vi "Weigth-Voltage.vi"() -> ()   [LabVIEW 2015]
uses:
  <vilib>/Utility/error.llb/DialogType.ctl
  <vilib>/DAQmx/read.llb/DAQmx Read (Analog DBL 1Chan 1Samp).vi
  <vilib>/DAQmx/create/channels.llb/DAQmx Create Channel (AI-Voltage-Basic).vi
  <vilib>/DAQmx/miscellaneous.llb/DAQmx Fill In Error Info.vi
panel:
  out "Peso[g]":dbl
  out "Waveform Chart":dbl(graph)
  out "Vi":dbl=0.7398038924745398 format="%0.2f"
  in  "stop":bool
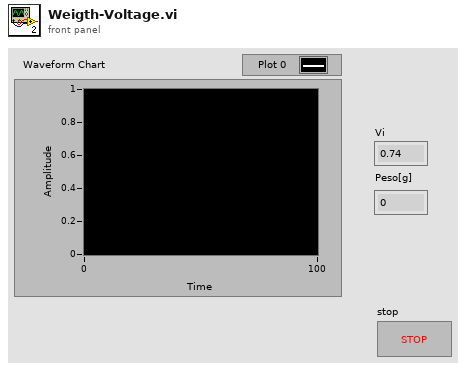
[diagram p1: front panel]
types:
  T1 = typedef "DialogType.ctl" = u16
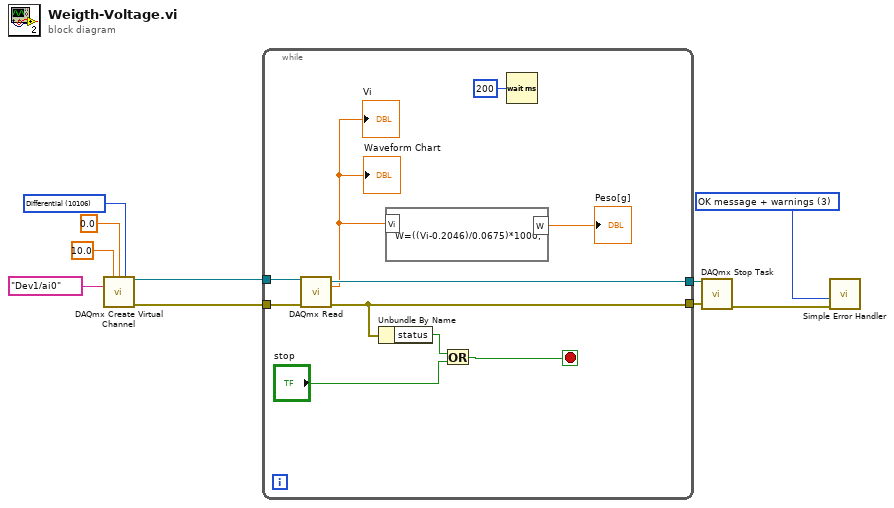
[diagram p0: block diagram]
diagram:
  w1 = 10106 items=["Default"=-1, "RSE"=10083, "NRSE"=10078, "Differential"=10106, "Pseudodifferential"=12529] ("input terminal configuration")
  w2 = T1 3 items=["no dialog", "OK message", "continue or stop message", "OK message + warnings", "continue/stop + warnings"] ("type of dialog (OK msg:1)")
  n1 = call-poly <vilib>:"DAQmx Create Virtual Channel.vi"("maximum value"=10.0, "minimum value"=0.0, "input terminal configuration"=w1, "physical channels"=tag "Dev1/ai0") -> ("task out"=w7:refnum<k21>, "error out"=w6:errorcluster)  [unwired: 10 in]
  n2 = while {
    tunnel: w7 -> [w20]
    tunnel: w6 -> [w19]
    tunnel: [w18] -> w5
    tunnel: [w14] -> w4
    stop <- w15 stop-if-true
    n3 = call-poly <vilib>:"DAQmx Read.vi"("task/channels in"=w20, "error in"=w19) -> ("task out"=w14:refnum<k21>, "data"=w12:dbl, "error out"=w18:errorcluster)  [unwired: 11 in]
    "Vi" <- w12
    "Waveform Chart" <- w12
    n4 = Unbundle By Name(w18) -> ("status"=w17:bool)
    n5 = formula code="W=((Vi-0.2046)/0.0675)*1000;"("Vi"=w12) -> ("W"=→"Peso[g]":dbl)
    n6 = Or(x=w17, y="stop") -> (x .or. y?=w15:bool)
    n7 = Wait (ms)(milliseconds to wait=u32 200) -> ()  [unwired: 1 out]
  }
  n8 = call <vilib>:"DAQmx Stop Task.vi"("task/channels in"=w4, "error in"=w5) -> ("error out"=w3:errorcluster)  [unwired: 12 in, 1 out]
  n9 = call <vilib>:"Simple Error Handler.vi"("type of dialog (OK msg:1)"=w2, "error in (no error)"=w3) -> ()  [unwired: 3 in, 5 out]
